vi "Get one Math Word design.vi"(8 "error in (no error)":errorcluster, 10 "reload MathCAD":bool, 11 "Design Inputs":T6) -> (0 "error out":errorcluster, 1 "Design Inputs":T4={"Q.Plant"=0.005, "C.CoagDoseMax"=0.01, "C.CoagStock"=0.01, "Ti.CoagStock"=0.0015, "EN.DrillSeries"=enum."English", "EN.TubeSeries"=enum."English", "N.SedTanks"=10.0, "N.SedBaysEst"=120.0, "W.SedPlate"=0.01, "L.SedPlateSheet"=0.0, "T.SedPlate"=10031039.999999998, "T.PlantWall"=0.03, "H.FlocOption"=0.01, "T.FlocBaffleRigidH"=1.7999999999999998, "T.ConcreteMin"=0.3, "T.SedWeir"=0.04, "T.FlocBaffleRigidV"=108000.0} {"T.FlocBaffleRigidV" min=0.0 max=0.2 step=0.001 format="%#.1f"; "T.SedWeir" min=0.001 max=0.2 step=0.001 format="%#.1f"; "T.SedPlate" min=0.001 max=0.05 step=0.001 format="%#.1f"; "T.FlocBaffleRigidH" min=0.0 max=0.2 step=0.001 format="%#.1f"; "T.ConcreteMin" min=0.005 max=0.2 step=0.001 format="%#.1f"; "L.SedPlateSheet" min=0.3 max=8.0 step=0.01 format="%#.1f"; "N.SedBaysEst" min=1.0 max=20.0 step=1.0 format="%#.0f"; "N.SedTanks" min=1.0 max=20.0 step=1.0 format="%#.0f"; "Ti.CoagStock" min=43200.0 max=360000.0 step=3600.0 format="%#.1f"; "H.FlocOption" min=0.5 max=4.0 step=0.01 format="%#.2f"; "C.CoagStock" min=50.0 max=500.0 step=1.0 format="%#.0f"; "C.CoagDoseMax" min=0.03 max=0.2 step=0.005 format="%#.0f"; "Q.Plant" min=0.001 max=0.2 step=0.0001 format="%#.1f"; "T.PlantWall" min=0.05 max=0.5 step=0.001 format="%#.1f"; "W.SedPlate" min=0.5 max=3.0 step=0.001 format="%#.1f"}, 2 "Project inputs":T3, 3 "User Information":T1 {"Country" items=["Afghanistan", "Aland Islands", "Albania", "Algeria", "American Samoa", "Andorra", "Angola", "Anguilla", "Antarctica", "Antigua And Barbuda", "Argentina", "Armenia", "Aruba", "Australia", "Austria", "Azerbaijan", "Bahamas", "Bahrain", "Bangladesh", "Barbados", "Belarus", "Belgium", "Belize", "Benin", "Bermuda", "Bhutan", "Bolivia", "Bosnia And Herzegovina", "Botswana", "Bouvet Island", "Brazil", "British Indian Ocean Territory", "Brunei Darussalam", "Bulgaria", "Burkina Faso", "Burundi", "Cambodia", "Cameroon", "Canada", "Cape Verde", "Cayman Islands", "Central African Republic", "Chad", "Chile", "China", "Christmas Island", "Cocos (Keeling) Islands", "Colombia", "Comoros", "Congo", "Congo, The Democratic Republic Of The", "Cook Islands", "Costa Rica", "Cote D'Ivoire", "Croatia", "Cuba", "Cyprus", "Czech Republic", "Denmark", "Djibouti", "Dominica", "Dominican Republic", "Ecuador", "Egypt", "El Salvador", "Equatorial Guinea", "Eritrea", "Estonia", "Ethiopia", "Falkland Islands (Malvinas)", "Faroe Islands", "Fiji", "Finland", "France", "French Guiana", "French Polynesia", "French Southern Territories", "Gabon", "Gambia", "Georgia", "Germany", "Ghana", "Gibraltar", "Greece", "Greenland", "Grenada", "Guadeloupe", "Guam", "Guatemala", "Guernsey", "Guinea", "Guinea-Bissau", "Guyana", "Haiti", "Heard Island And Mcdonald Islands", "Holy See (Vatican City State)", "Honduras", "Hong Kong", "Hungary", "Iceland", "India", "Indonesia", "Iran, Islamic Republic Of", "Iraq", "Ireland", "Isle Of Man", "Israel", "Italy", "Jamaica", "Japan", "Jersey", "Jordan", "Kazakhstan", "Kenya", "Kiribati", "Korea, Democratic People'S Republic Of", "Korea, Republic Of", "Kuwait", "Kyrgyzstan", "Lao People'S Democratic Republic", "Latvia", "Lebanon", "Lesotho", "Liberia", "Libyan Arab Jamahiriya", "Liechtenstein", "Lithuania", "Luxembourg", "Macao", "Macedonia, The Former Yugoslav Republic Of", "Madagascar", "Malawi", "Malaysia", "Maldives", "Mali", "Malta", "Marshall Islands", "Martinique", "Mauritania", "Mauritius", "Mayotte", "Mexico", "Micronesia, Federated States Of", "Moldova, Republic Of", "Monaco", "Mongolia", "Montserrat", "Morocco", "Mozambique", "Myanmar", "Namibia", "Nauru", "Nepal", "Netherlands", "Netherlands Antilles", "New Caledonia", "New Zealand", "Nicaragua", "Niger", "Nigeria", "Niue", "Norfolk Island", "Northern Mariana Islands", "Norway", "Oman", "Pakistan", "Palau", "Palestinian Territory, Occupied", "Panama", "Papua New Guinea", "Paraguay", "Peru", "Philippines", "Pitcairn", "Poland", "Portugal", "Puerto Rico", "Qatar", "Reunion", "Romania", "Russian Federation", "Rwanda", "Saint Helena", "Saint Kitts And Nevis", "Saint Lucia", "Saint Pierre And Miquelon", "Saint Vincent And The Grenadines", "Samoa", "San Marino", "Sao Tome And Principe", "Saudi Arabia", "Senegal", "Serbia And Montenegro", "Seychelles", "Sierra Leone", "Singapore", "Slovakia", "Slovenia", "Solomon Islands", "Somalia", "South Africa", "South Georgia And The South Sandwich Islands", "Spain", "Sri Lanka", "Sudan", "Suriname", "Svalbard And Jan Mayen", "Swaziland", "Sweden", "Switzerland", "Syrian Arab Republic", "Taiwan, Province Of China", "Tajikistan", "Tanzania, United Republic Of", "Thailand", "Timor-Leste", "Togo", "Tokelau", "Tonga", "Trinidad And Tobago", "Tunisia", "Turkey", "Turkmenistan", "Turks And Caicos Islands", "Tuvalu", "Uganda", "Ukraine", "United Arab Emirates", "United Kingdom", "United States", "United States Minor Outlying Islands", "Uruguay", "Uzbekistan", "Vanuatu", "Venezuela", "Viet Nam", "Virgin Islands, British", "Virgin Islands, U.S.", "Wallis And Futuna", "Western Sahara", "Yemen", "Zambia", "Zimbabwe", "(Not Specified)"]}, 4 "ADT Commands":T5, 5 "Revision":i32, 6 "Success":bool, 7 "SVN Checkout output":string, 9 "Find-Replace":cluster{"Find":string, "Replace":string}[](array[cluster]))   [LabVIEW 2015]
uses:
  mathcad/Simple/MathCAD cmd.ctl
  Project commands.ctl
  AguaClara Library.lvlib
  <vilib>/Utility/SMTP/NI_SMTPEmail.lvlib
  Word cmd.ctl
  Project inputs.ctl
  User Information.ctl
  Basic Inputs.ctl
  ADT Commands.ctl
  packed var.ctl
  Country Ring.ctl
panel:
  in  "Tab Control":enum32{"Page 1", "Page 2", "Page 3"}(tab)
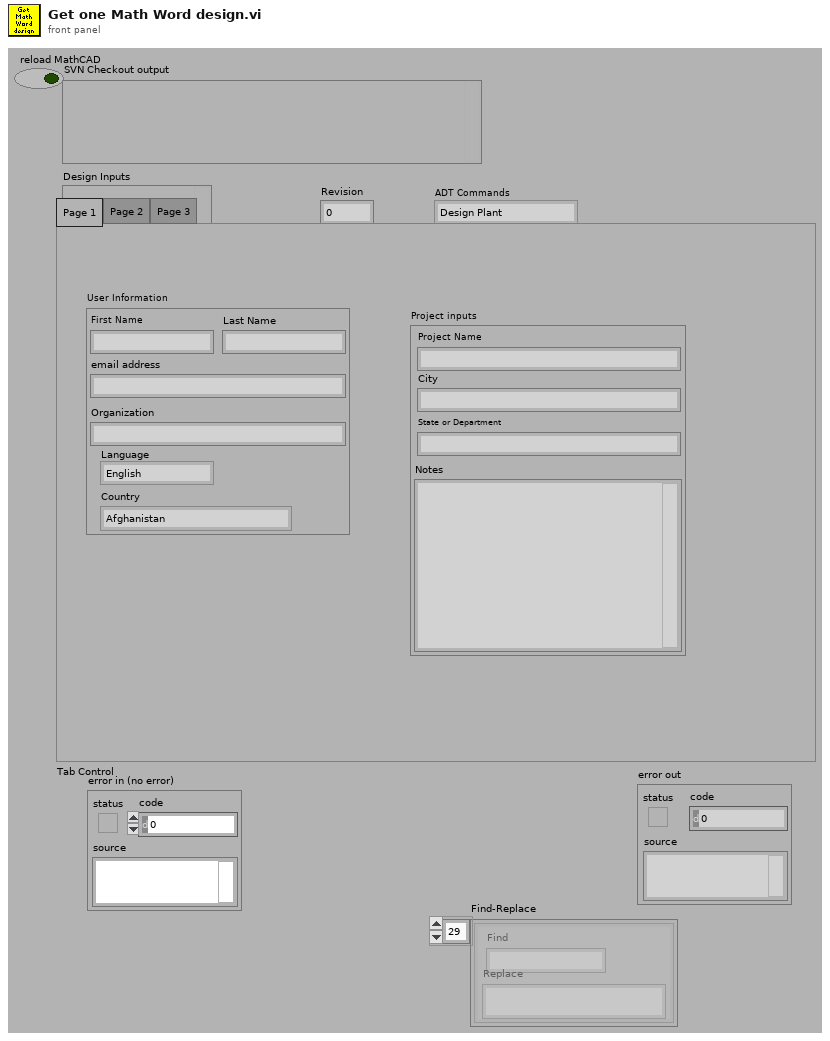
[diagram p1: front panel]
types:
  T1 = typedef "AguaClara Library.lvlib/User Information.ctl" = cluster{"First Name":string, "Last Name":string, "Email Address":string, "Organization":string, "Language":enum16{"English", "Español", "French"}, "Country":T2}
  T2 = typedef "Country Ring.ctl" = u16
  T3 = typedef "AguaClara Library.lvlib/Project inputs.ctl" = cluster{"Project Name":string, "City":string, "State":string, "Notes":string}
  T4 = typedef "AguaClara Library.lvlib/Basic Inputs.ctl" = cluster{"Q.Plant":dbl[unit], "C.CoagDoseMax":dbl[unit], "C.CoagStock":dbl[unit], "Ti.CoagStock":dbl[unit], "EN.DrillSeries":enum16{"English", "Metric"}, "EN.TubeSeries":enum16{"English", "Metric"}, "N.SedTanks":dbl, "N.SedBaysEst":dbl, "W.SedPlate":dbl[unit], "L.SedPlateSheet":dbl[unit], "T.SedPlate":dbl[unit], "T.PlantWall":dbl[unit], "H.FlocOption":dbl[unit], "T.FlocBaffleRigidH":dbl[unit], "T.ConcreteMin":dbl[unit], "T.SedWeir":dbl[unit], "T.FlocBaffleRigidV":dbl[unit]}
  T5 = typedef "ADT Commands.ctl" = enum16{"Design Plant", "CheckOut MathCAD Files", "Restart"}
  T6 = typedef "packed var.ctl" = variant
  T7 = typedef "user project design.ctl" = cluster{"Key":string[], "Value":string[]}
  T8 = typedef "AguaClara Library.lvlib/Word cmd.ctl" = enum16{"Initialize", "Load User Inputs", "Update Fields", "Replace Variables", "Save pdf", "Close Word"}
  T9 = typedef "MathCAD cmd.ctl" = enum16{"Open App", "Open Worksheet", "Close Worksheet", "Load Variable Ref", "Send Number", "Send Cluster", "Send Array", "Send String", "Calculate", "Get MathCAD data", "Close MathCAD"}
  T10 = typedef "AguaClara Library.lvlib/Project commands.ctl" = enum16{"Load base file", "Load User", "Read paths", "Open Project", "New project", "Edit project", "Delete project", "Mail project", "save design", "open design"}
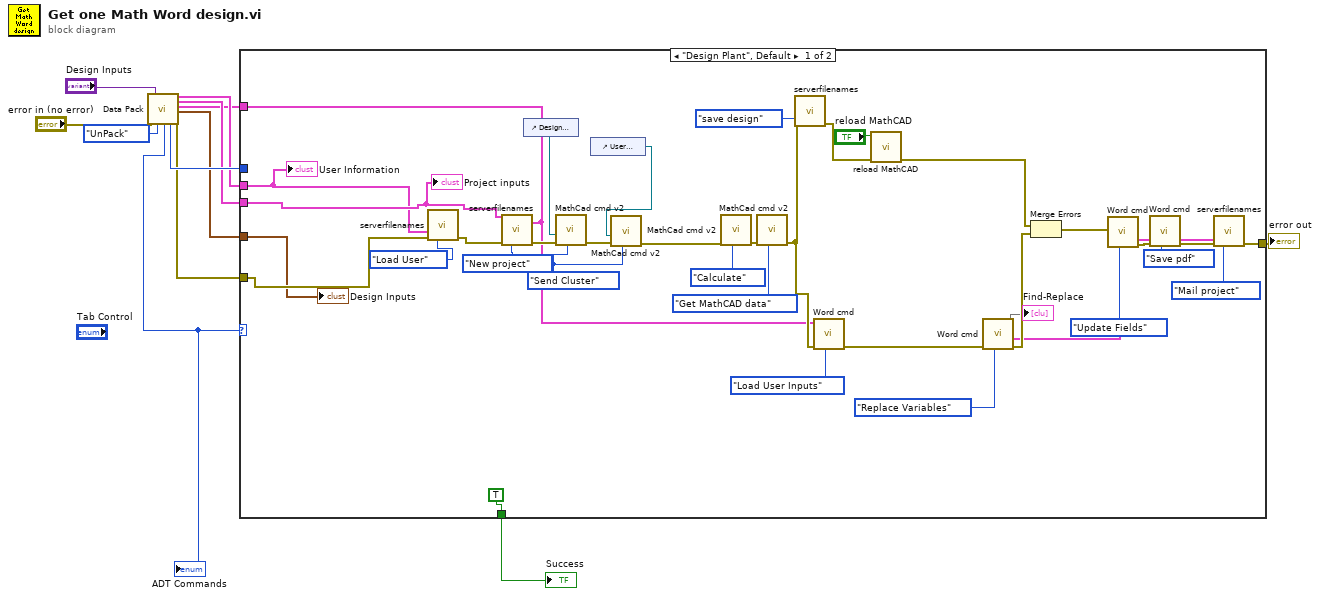
[diagram p0: block diagram]
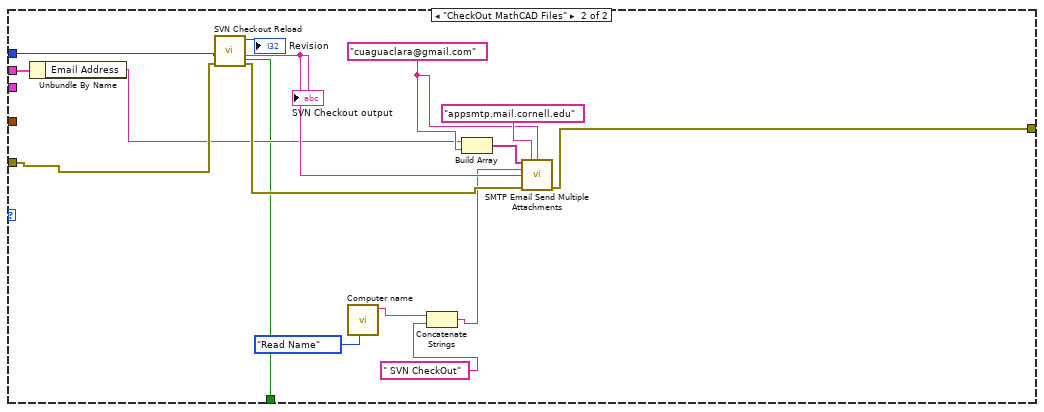
[diagram p2: hidden frame]
diagram:
  n1 = call "Data Pack.vi"("error in"="error in (no error)", "Packed In"="Design Inputs", "Data transform"=enum16{"Pack", "UnPack"}."UnPack") -> ("ADT Commands out"=w8:T5, "ADT version out"=w7:i32, "User Information out"=w6:T1, "Project Info out"=w5:T3, "user project design"=w1:T7, "Design Inputs out"=w4:T4, "error out"=w3:errorcluster)  [unwired: 9 in, 1 out]
  "ADT Commands" <- w8
  n2 = case shown="\"Design Plant\", Default" w8 {
    tunnel: [w45 w59] -> w12
    tunnel: w4 -> [w34 _]
    tunnel: w6 -> [w31 w56]
    tunnel: w5 -> [w40 _]
    tunnel: w7 -> [_ w64]
    tunnel: w3 -> [w36 w57]
    tunnel: [TRUE ("Success") w53] -> w2
    tunnel: w1 -> [w19 _]
    frame "Design Plant", Default {
      w16 = MathCAD_cmd."Send Cluster" ("MathCAD cmds")
      n3 = call "serverfilenames.vi"("User Information"=w31, "error in (no error)"=w36, "Project command"=Project_commands."Load User") -> ("error out"=w48:errorcluster)  [unwired: 8 in, 4 out]
      n4 = call "serverfilenames.vi"("Project Info"=w40, "Project Design Expert"=w19, "error in (no error)"=w48, "Project command"=Project_commands."New project") -> ("error out"=w41:errorcluster)  [unwired: 7 in, 4 out]
      n5 = control-ref of="Design Inputs"() -> (w42:refnum<vi>)
      n6 = call "MathCad cmd v2.vi"("MathCAD cmds"=w16, "error in"=w41, "Clust Refnum"=w42) -> ("first error out"=w17:errorcluster)  [unwired: 7 in, 1 out]
      n7 = control-ref of="User Information"() -> (w15:refnum<vi>)
      n8 = call "MathCad cmd v2.vi"("MathCAD cmds"=w16, "error in"=w17, "Clust Refnum"=w15) -> ("first error out"=w14:errorcluster)  [unwired: 7 in, 1 out]
      n9 = call "MathCad cmd v2.vi"("MathCAD cmds"=MathCAD_cmd."Calculate", "error in"=w14) -> ("first error out"=w38:errorcluster)  [unwired: 8 in, 1 out]
      n10 = call "MathCad cmd v2.vi"("MathCAD cmds"=MathCAD_cmd."Get MathCAD data", "error in"=w38) -> ("first error out"=w25:errorcluster)  [unwired: 8 in, 1 out]
      n11 = call "serverfilenames.vi"("error in (no error)"=w25, "Project command"=Project_commands."save design") -> ("error out"=w22:errorcluster)  [unwired: 9 in, 4 out]
      n12 = call "Word cmd.vi"("Word cmd"=Word_cmd."Load User Inputs", "Error In (no error)"=w25, "DesignRequest"=w19) -> ("error out"=w32:errorcluster)  [unwired: 7 in, 1 out]
      n13 = call "reload MathCAD.vi"("error in"=w22, "reload"="reload MathCAD") -> ("error out"=w21:errorcluster)  [unwired: 9 in]
      n14 = call "Word cmd.vi"("Word cmd"=Word_cmd."Replace Variables", "Error In (no error)"=w32) -> ("error out"=w24:errorcluster, "Find-Replace"=w18:cluster{"Find":string, "Replace":string}[], 3:→"Find-Replace")  [unwired: 7 in]
      n15 = Merge Errors(w21, w24) -> (w23:errorcluster)
      n16 = call "Word cmd.vi"("Word cmd"=Word_cmd."Update Fields", "Error In (no error)"=w23) -> ("error out"=w27:errorcluster)  [unwired: 8 in, 1 out]
      n17 = call "Word cmd.vi"("Word cmd"=Word_cmd."Save pdf", "Error In (no error)"=w27) -> ("error out"=w28:errorcluster)  [unwired: 8 in, 1 out]
      n18 = call "serverfilenames.vi"("error in (no error)"=w28, "Project command"=Project_commands."Mail project", "Good design"=w18) -> ("error out"=w45:errorcluster)  [unwired: 8 in, 4 out]
      "Project inputs" <- w40
      "User Information" <- w31
      "Design Inputs" <- w34
    }
    frame "CheckOut MathCAD Files" {
      w61 = "cuaguaclara@gmail.com" ("return address")
      n19 = Unbundle By Name(w56) -> ("Email Address"=w55:string)
      n20 = call "SVN Checkout Reload.vi"("error in"=w57, "ADT version"=w64) -> ("error out"=w60:errorcluster, "SVN Checkout output"=w58:string, "Revision"=→"Revision":i32, "Success"=w53:bool)  [unwired: 4 in, 2 out]
      "SVN Checkout output" <- w58
      n21 = call "Computer name.vi"("cmd"=enum16{"Load Name", "Read Name"}."Read Name") -> ("Computer name"=w51:string)  [unwired: 9 in, 1 out]
      n22 = Concatenate Strings(w51, " SVN CheckOut" ("subject ([No Subject])")) -> (w49:string)
      n23 = Build Array(w55, w61) -> (w63:string[])
      n24 = call <vilib>:"SMTP Email Send Multiple Attachments.vi"("recipients"=w63, "mail server"="appsmtp.mail.cornell.edu", "return address"=w61, "subject ([No Subject])"=w49, "message"=w58, "error in (no error)"=w60) -> ("error out"=w59:errorcluster)  [unwired: 8 in, 1 out]
    }
  }
  "error out" <- w12
  "Success" <- w2
